vi "曲线处理.vi"(0 "上限":sgl, 1 "下限":sgl, 2 "起点":dbl, 3 "终点":dbl, 4 "历史数据":sgl[](array[numeric])) -> (5 "值":sgl, 6 "值显示":string, 7 "曲线数组":sgl[](array[numeric]), 10 "范围内?":bool)   [LabVIEW 2018]
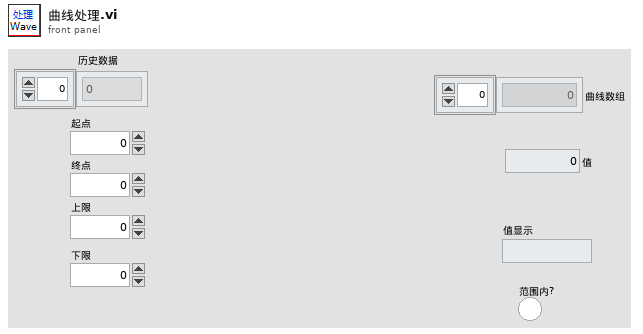
[diagram p1: front panel]
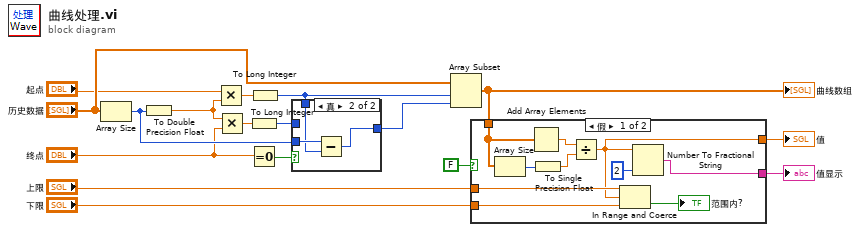
[diagram p0: block diagram]
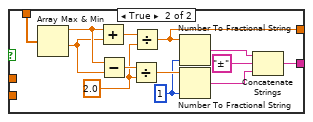
[diagram p2: hidden frame]
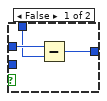
[diagram p3: hidden frame]
diagram:
  n1 = Array Size(array="历史数据") -> (size(s)=w10:i32)
  n2 = To Double Precision Float(number=w10) -> (double precision float=w5:dbl)
  n3 = Multiply(x="起点", y=w5) -> (x*y=w12:dbl)
  n4 = Multiply(x=w5, y="终点") -> (x*y=w11:dbl)
  n5 = To Long Integer(number=w11) -> (32bit integer=w8:i32)
  n6 = Equal To 0?(x="终点") -> (x = 0?=w17:bool)
  n7 = To Long Integer(number=w12) -> (32bit integer=w7:i32)
  n8 = case shown="真" w17 {
    tunnel: w10 -> [_ w23]
    tunnel: w8 -> [w20 _]
    tunnel: w7 -> [w19 w22]
    tunnel: [w18 w21] -> w6
    frame False {
      n9 = Subtract(x=w20, y=w19) -> (x-y=w18:i32)
    }
    frame True {
      n10 = Subtract(x=w23, y=w22) -> (x-y=w21:i32)
    }
  }
  n11 = Array Subset(array="历史数据", index=w7, length=w6) -> (w14:sgl[])
  "曲线数组" <- w14
  n12 = case shown="假" FALSE {
    tunnel: w14 -> [w33 w46]
    tunnel: [w28 w35] -> w16
    tunnel: "上限" -> [w26 _]
    tunnel: "下限" -> [w25 _]
    tunnel: [w24 w34] -> w13
    frame False {
      n13 = Array Size(array=w33) -> (size(s)=w31:i32)
      n14 = Add Array Elements(numeric array=w33) -> (sum=w32:sgl)
      n15 = To Single Precision Float(number=w31) -> (single precision float=w30:sgl)
      n16 = Divide(x=w32, y=w30) -> (x/y=w24:sgl)
      n17 = In Range and Coerce(upper limit=w26, x=w24, lower limit=w25) -> (In Range?=→"范围内?":bool)  [unwired: 1 out]
      n18 = Number To Fractional String(number=w24, precision (6)=i16 2 ("精度(6)")) -> (F-format string=w28:string)  [unwired: 2 in]
    }
    frame True {
      w39 = i16 1 ("精度(6)")
      w41 = sgl 2.0
      n19 = Array Max & Min(array=w46) -> (max value=w44:sgl, min value=w43:sgl)  [unwired: 2 out]
      n20 = Add(x=w44, y=w43) -> (x+y=w45:sgl)
      n21 = Subtract(x=w44, y=w43) -> (x-y=w42:sgl)
      n22 = Divide(x=w42, y=w41) -> (x/y=w40:sgl)
      n23 = Divide(x=w45, y=w41) -> (x/y=w34:sgl)
      n24 = Number To Fractional String(number=w34, precision (6)=w39) -> (F-format string=w38:string)  [unwired: 2 in]
      n25 = Number To Fractional String(number=w40, precision (6)=w39) -> (F-format string=w36:string)  [unwired: 2 in]
      n26 = Concatenate Strings(w38, "±", w36) -> (w35:string)
    }
  }
  "值显示" <- w16
  "值" <- w13
